vi "Configure Flow.vi"(6 "Flow Measurement Multiplied Adjustment (1)":dbl=1.0, 7 "Flow Measurement Added Adjustment (0)":dbl, 8 "error in (no error)":errorcluster, 9 "Flow Stability Value (0.1)":dbl=0.1, 10 "Flow Stability Units (0: Flow Units/Sec)":u16(ring) items=["Flow Units/Sec", "Percentage of Active Molbloc"], 11 "VISA resource name":refnum<visa-resource-name>) -> (0 "error out":errorcluster, 3 "VISA resource name out":refnum<visa-resource-name>)   [LabVIEW 2023, in "Fluke Molbox 1 Plus.lvlib"]
doc: "Configures aspects of the instrument that deal with flow. This includes setting the flow stability and the adjustment used for flow measurements."
uses:
  Fluke Molbox 1 Plus.lvlib
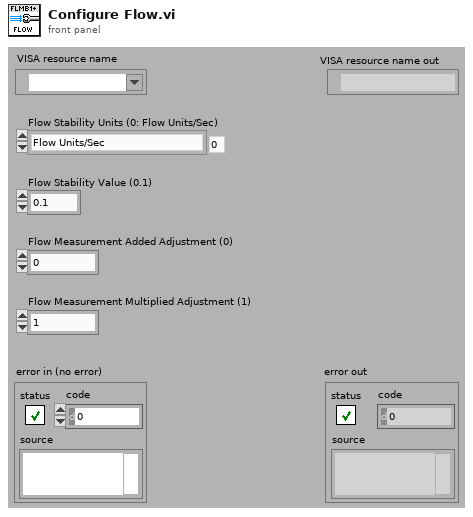
[diagram p1: front panel]
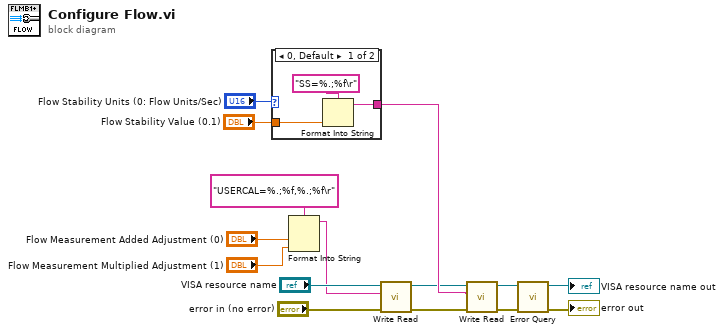
[diagram p0: block diagram]
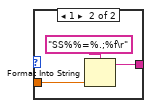
[diagram p2: hidden frame]
diagram:
  n1 = case shown="0, Default" "Flow Stability Units (0: Flow Units/Sec)" {
    tunnel: "Flow Stability Value (0.1)" -> [w18 w21]
    tunnel: [w16 w19] -> w10
    frame 0, Default {
      n2 = Format Into String(format string="SS=%.;%f\r", w18) -> (resulting string=w16:string)  [unwired: 2 in, 1 out]
    }
    frame 1 {
      n3 = Format Into String(format string="SS%%=%.;%f\r", w21) -> (resulting string=w19:string)  [unwired: 2 in, 1 out]
    }
  }
  n4 = Format Into String(format string="USERCAL=%.;%f,%.;%f\r", "Flow Measurement Added Adjustment (0)", "Flow Measurement Multiplied Adjustment (1)") -> (resulting string=w8:string)  [unwired: 2 in, 1 out]
  n5 = call "Write Read.vi"("error in (no error)"="error in (no error)", "Write String"=w8, "VISA resource name"="VISA resource name") -> ("error out"=w6:errorcluster, "VISA resource name out"=w5:refnum<visa-resource-name>)  [unwired: 6 in, 1 out]
  n6 = call "Write Read.vi"("error in (no error)"=w6, "Write String"=w10, "VISA resource name"=w5) -> ("error out"=w3:errorcluster, "VISA resource name out"=w4:refnum<visa-resource-name>)  [unwired: 6 in, 1 out]
  n7 = call "Error Query.vi"("error in (no error)"=w3, "VISA resource name"=w4) -> ("error out"=→"error out":errorcluster, "VISA resource name out"=→"VISA resource name out":refnum<visa-resource-name>)  [unwired: 6 in, 2 out]
